vi "Dialog_Enter Stage Position.vi"(8 "Error In":errorcluster) -> (0 "Error Out":errorcluster, 2 "Cancelled?":bool, 3 "Macro Commands":T2)   [LabVIEW 2012]
uses:
  Custom Controls and Typedefs/Macro_CommandStruct.ctl
  Custom Controls and Typedefs/Macro_Action_List.ctl
  Custom Controls and Typedefs/Macro_ArgumentStruct.ctl
  Custom Controls/Stage Position Data.ctl
  Dialog_Enter Stage Position_UI Refnums.ctl
  GFG/GFG library.lvlib
panel:
  in  "Stage Position Data":T1 caption="Current Position"
  in  "Cancel Button":bool
  in  "OK Button":bool
  in  "PSM_Table":string[][](table)
  in  "Position Entry Mode":T5(radio)
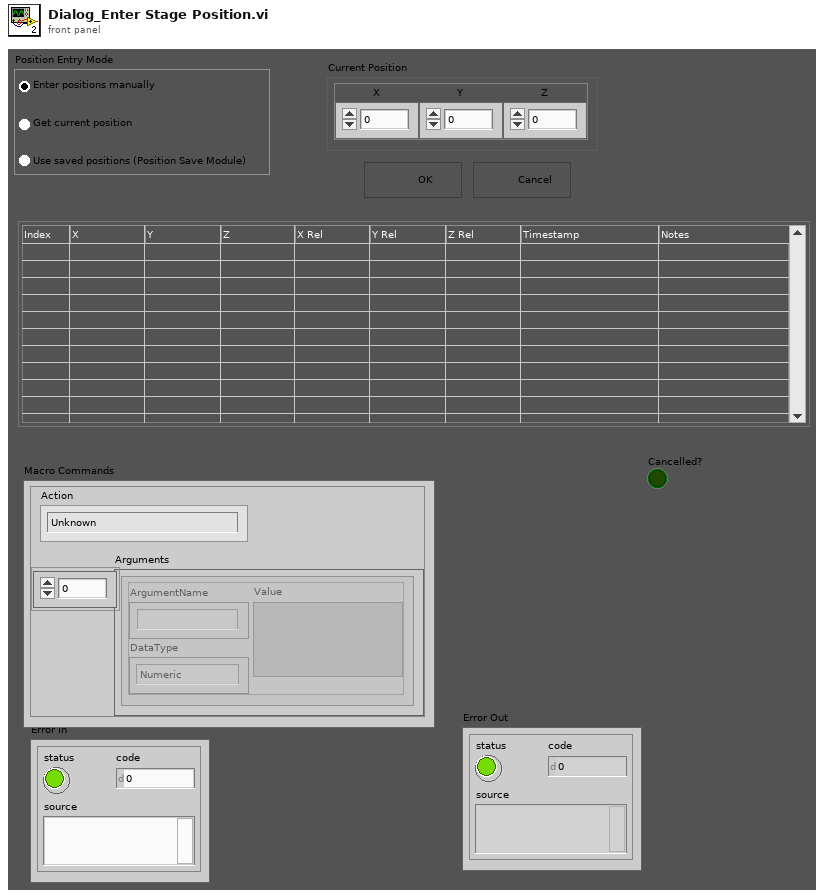
[diagram p1: front panel]
types:
  T1 = typedef "Stage Position Data.ctl" = cluster{"X":dbl, "Z":dbl, "Y":dbl}
  T2 = typedef "Macro_CommandStruct.ctl" = cluster{"Action":T3, "Arguments":T4[]}
  T3 = typedef "Macro_Action_List.ctl" = enum16{"Unknown", "2D.Frame.Scan", "2D.Line.Scan", "Load.Settings.File", "Move.To.Position", "Pause", "Z.Stack", "LOOP.Start", "LOOP.End"}
  T4 = typedef "Macro_ArgumentStruct.ctl" = cluster{"ArgumentName":string, "DataType":enum16{"Numeric", "String"}, "Value":variant}
  T5 = enum32{"Enter positions manually", "Get current position", "Use saved positions (Position Save Module)"}
  T6 = enum8{"Enabled", "Disabled", "Disabled and Grayed Out"}
  T7 = typedef "Dialog_Enter Stage Position_UI Refnums.ctl" = cluster{"PSM Table":refnum<vi>, "Stop Button":refnum<vi>, "Stage Position":refnum<vi>}
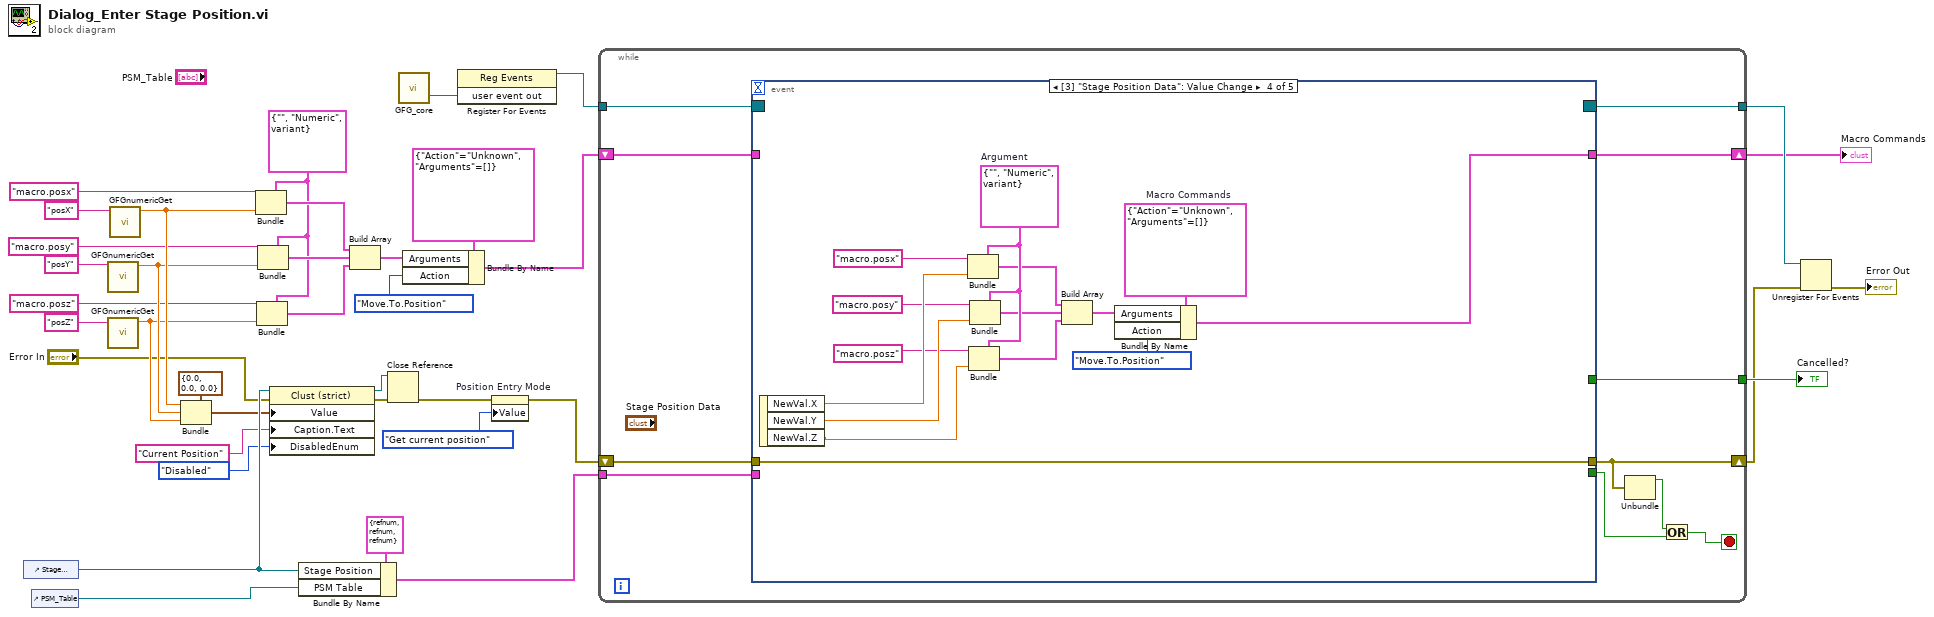
[diagram p0: block diagram]
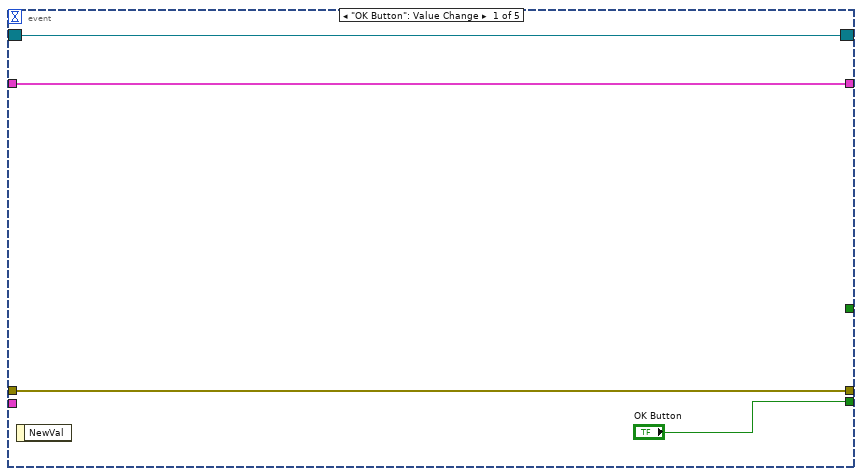
[diagram p2: hidden frame]
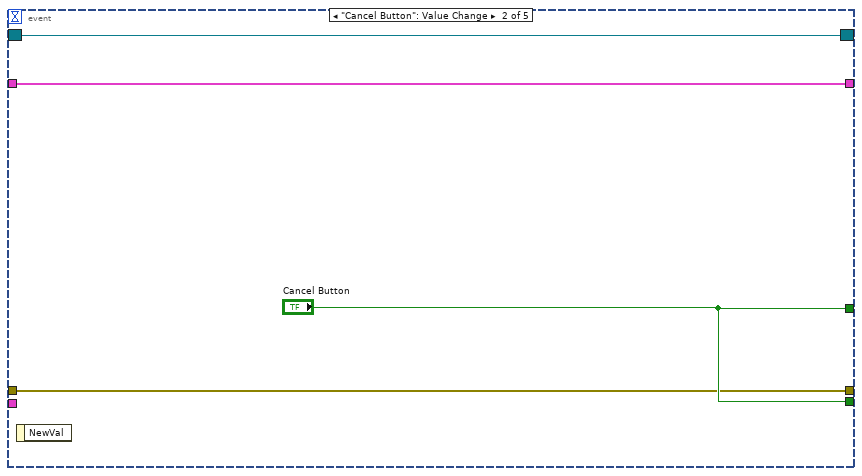
[diagram p3: hidden frame]
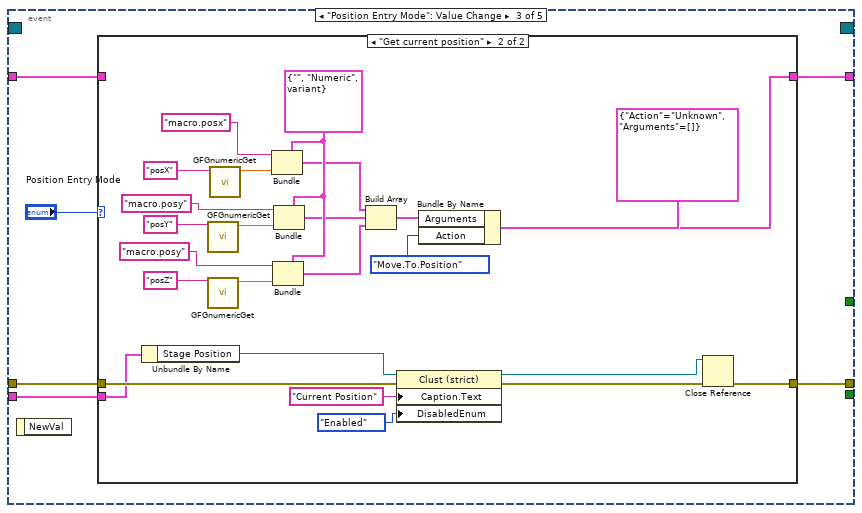
[diagram p4: hidden frame]
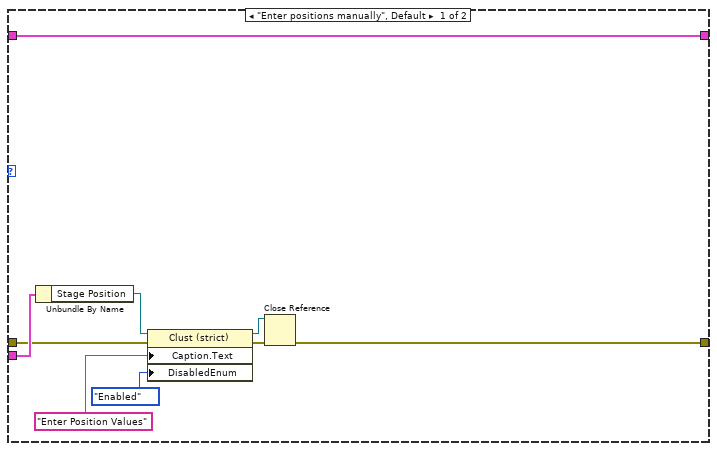
[diagram p5: hidden frame]
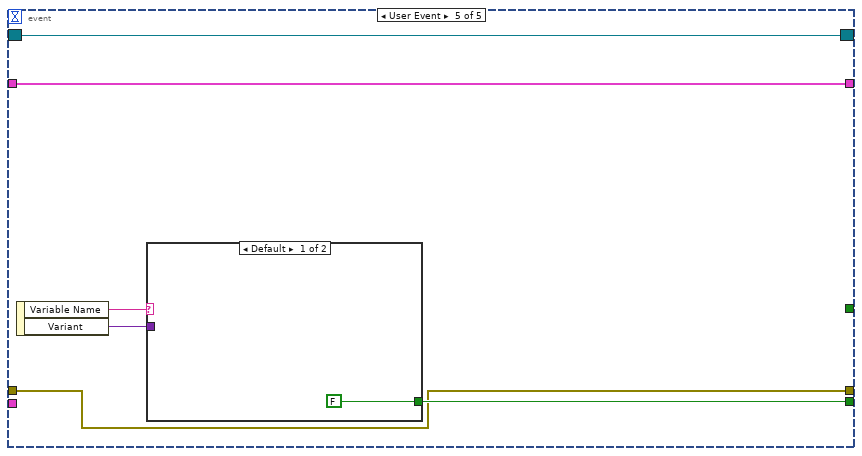
[diagram p6: hidden frame]
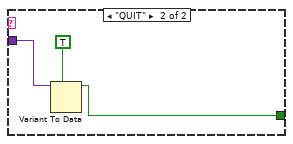
[diagram p7: hidden frame]
diagram:
  w26 = T4 {"ArgumentName"="", "DataType"=enum."Numeric", "Value"=variant} ("Argument")
  n1 = control-ref of="Stage Position Data"() -> (w13:refnum<vi>)
  n2 = control-ref of="PSM_Table"() -> (w20:refnum<vi>)
  n3 = call "GFGnumericGet.vi"("Variable Name in"="posY") -> ("Numeric"=w16:dbl)  [unwired: 9 in, 1 out]
  n4 = call "GFGnumericGet.vi"("Variable Name in"="posZ") -> ("Numeric"=w15:dbl)  [unwired: 9 in, 1 out]
  n5 = call "GFGnumericGet.vi"("Variable Name in"="posX") -> ("Numeric"=w17:dbl)  [unwired: 9 in, 1 out]
  n6 = Bundle(cluster=T1 {"X"=0.0, "Z"=0.0, "Y"=0.0} ("Stage Position Data"), "X"=w17, "Z"=w16, "Y"=w15) -> (w10:T1)
  n7 = Bundle(cluster=w26, "ArgumentName"="macro.posx" ("Variable Name in"), "Value"=w17) -> (w27:T4)  [unwired: 1 in]
  n8 = Bundle(cluster=w26, "ArgumentName"="macro.posz" ("Variable Name in"), "Value"=w15) -> (w29:T4)  [unwired: 1 in]
  n9 = Bundle(cluster=w26, "ArgumentName"="macro.posy" ("Variable Name in"), "Value"=w16) -> (w28:T4)  [unwired: 1 in]
  n10 = property class="Clust (strict)"(reference=w13, error in="Error In", "Value"=w10, "Caption.Text"="Current Position" ("Label.Text"), "DisabledEnum"=T6."Disabled" ("Disabled")) -> (reference out=w6:refnum<vi>, error out=w7:errorcluster)
  n11 = Bundle By Name(cluster=T7 {"PSM Table"=refnum, "Stop Button"=refnum, "Stage Position"=refnum} ("Record Stage Position_UI Refnums"), "Stage Position"=w13, "PSM Table"=w20) -> (w34:T7)
  n12 = Build Array(w27, w28, w29) -> (w31:T4[])
  n13 = Close Reference(reference=w6, error in (no error)=w7) -> (error out=w5:errorcluster)
  n14 = call "GFG_core.vi"() -> ("user event out"=w38:refnum<user-event>)  [unwired: 13 in, 6 out]
  n15 = Bundle By Name(cluster=T2 {"Action"=enum."Unknown", "Arguments"=[]} ("Macro Commands"), "Arguments"=w31, "Action"=Macro_Action_List."Move.To.Position") -> (w22:T2)
  n16 = register-events(w38) -> (reference out=w37:refnum<event-registration>)  [unwired: 2 in, 1 out]
  n17 = property on="Position Entry Mode" class="RadioBtnsControl (strict)"(error in=w5, "Value"=T5."Get current position" ("Position Entry Mode")) -> (error out=w19:errorcluster)  [unwired: 1 in, 1 out]
  n18 = while {
    tunnel: w37 -> [w49]
    tunnel: [w48] -> w36
    tunnel: w34 -> [w47]
    tunnel: [w46] -> w33
    shift-right: [w45] -> w21
    shift-left: w22 -> [w44]
    shift-right: [w43] -> w14
    shift-left: w19 -> [w39]
    stop <- w40 stop-if-true
    n19 = event shown="[3] \"Stage Position Data\": Value Change" {
      selector: w49 -> [w53 w56 _ _ w115]
      dyn-events: [w53 w56 _ _ w115] -> w48
      timeout: _ -> [_ _ _ _ _]
      tunnel: ["OK Button" "Cancel Button" _ _ w116] -> w42
      tunnel: w47 -> [_ _ w59 _ _]
      tunnel: [_ "Cancel Button" _ _ _] -> w46
      tunnel: [w51 w55 w62 w106 w114] -> w45
      tunnel: w44 -> [w51 w55 w61 _ w114]
      tunnel: w39 -> [w50 w54 w60 w105 w113]
      tunnel: [w50 w54 w58 w105 w113] -> w43
      event "OK Button": Value Change {
        n20 = event-data() -> ()  [unwired: 1 in, 1 out]
      }
      event "Cancel Button": Value Change {
        n21 = event-data() -> ()  [unwired: 1 in, 1 out]
      }
      event "Position Entry Mode": Value Change {
        n22 = event-data() -> ()  [unwired: 1 in, 1 out]
        n23 = case shown="\"Get current position\"" "Position Entry Mode" {
          tunnel: [w72 w85] -> w62
          tunnel: w61 -> [w72 _]
          tunnel: w60 -> [w65 w79]
          tunnel: w59 -> [w71 w78]
          tunnel: [w64 w77] -> w58
          frame "Enter positions manually", Default {
            n24 = Unbundle By Name(w71) -> ("Stage Position"=w68:refnum<vi>)
            n25 = property class="Clust (strict)"(reference=w68, error in=w65, "Caption.Text"="Enter Position Values" ("Label.Text"), "DisabledEnum"=T6."Enabled" ("Disabled")) -> (reference out=w70:refnum<vi>, error out=w69:errorcluster)
            n26 = Close Reference(reference=w70, error in (no error)=w69) -> (error out=w64:errorcluster)
          }
          frame "Get current position" {
            w92 = T4 {"ArgumentName"="", "DataType"=enum."Numeric", "Value"=variant} ("Argument")
            n27 = Unbundle By Name(w78) -> ("Stage Position"=w82:refnum<vi>)
            n28 = call "GFGnumericGet.vi"("Variable Name in"="posY") -> ("Numeric"=w94:dbl)  [unwired: 9 in, 1 out]
            n29 = call "GFGnumericGet.vi"("Variable Name in"="posZ") -> ("Numeric"=w91:dbl)  [unwired: 9 in, 1 out]
            n30 = call "GFGnumericGet.vi"("Variable Name in"="posX") -> ("Numeric"=w96:dbl)  [unwired: 9 in, 1 out]
            n31 = Bundle(cluster=w92, "ArgumentName"="macro.posx" ("Variable Name in"), "Value"=w96) -> (w90:T4)  [unwired: 1 in]
            n32 = Bundle(cluster=w92, "ArgumentName"="macro.posy" ("Variable Name in"), "Value"=w91) -> (w88:T4)  [unwired: 1 in]
            n33 = Bundle(cluster=w92, "ArgumentName"="macro.posy" ("Variable Name in"), "Value"=w94) -> (w89:T4)  [unwired: 1 in]
            n34 = Build Array(w90, w89, w88) -> (w86:T4[])
            n35 = property class="Clust (strict)"(reference=w82, error in=w79, "Caption.Text"="Current Position" ("Label.Text"), "DisabledEnum"=T6."Enabled" ("Disabled")) -> (reference out=w84:refnum<vi>, error out=w83:errorcluster)
            n36 = Bundle By Name(cluster=T2 {"Action"=enum."Unknown", "Arguments"=[]} ("Macro Commands"), "Arguments"=w86, "Action"=Macro_Action_List."Move.To.Position") -> (w85:T2)
            n37 = Close Reference(reference=w84, error in (no error)=w83) -> (error out=w77:errorcluster)
          }
        }
      }
      event Value Change {
        w108 = T2 {"Action"=enum."Unknown", "Arguments"=[]}  # Macro Commands
        w112 = T4 {"ArgumentName"="", "DataType"=enum."Numeric", "Value"=variant}  # Argument
        n38 = event-data() -> ("NewVal.X"=w104:dbl, "NewVal.Y"=w103:dbl, "NewVal.Z"=w102:dbl)  [unwired: 1 in]
        n39 = Bundle(cluster=w112, "ArgumentName"="macro.posx" ("Variable Name in"), "Value"=w104) -> (w111:T4)  [unwired: 1 in]
        n40 = Bundle(cluster=w112, "ArgumentName"="macro.posz" ("Variable Name in"), "Value"=w102) -> (w109:T4)  [unwired: 1 in]
        n41 = Bundle(cluster=w112, "ArgumentName"="macro.posy" ("Variable Name in"), "Value"=w103) -> (w110:T4)  [unwired: 1 in]
        n42 = Build Array(w111, w110, w109) -> (w107:T4[])
        n43 = Bundle By Name(cluster=w108, "Arguments"=w107, "Action"=Macro_Action_List."Move.To.Position") -> (w106:T2)
      }
      event User Event {
        n44 = event-data() -> ("Variable Name"=w118:string, "Variant"=w117:variant)  [unwired: 1 in]
        n45 = case shown="Default" w118 {
          tunnel: w117 -> [_ w121]
          tunnel: [FALSE w120] -> w116
          frame Default {
          }
          frame "QUIT" {
            n46 = Variant To Data(type=TRUE, Variant=w121) -> (data=w120:bool)  [unwired: 1 in, 1 out]
          }
        }
      }
    }
    n47 = Unbundle(w43) -> ("status"=w41:bool)  [unwired: 2 out]
    n48 = Or(x=w41, y=w42) -> (x .or. y?=w40:bool)
  }
  "Cancelled?" <- w33
  "Macro Commands" <- w21
  n49 = Unregister For Events(event registration refnum=w36, error in=w14) -> (error out=→"Error Out":errorcluster)
